vi "Handler - Calib BeginFinish.vi"(8 "error in (no error)":errorcluster, 10 "Finish/Begin (Finish)":bool, 11 "Controller (Host) Data in":T1) -> (0 "error out":errorcluster, 3 "Controller (Host) Data out":T1)   [LabVIEW 2018]
uses:
  cRIO RT Comms/Private Controls/Stream Data.ctl
  cRIO RT Comms/cRIO RT Comms.lvlib
  Top Level/Shared Controls/cRIO State.ctl
  Private Controls/State.ctl
  Controller (Host).lvlib
  Public Controls/APU Select.ctl
  Public Controls/Login Access.ctl
  Private Controls/Controller (Host) Data.ctl
  Top Level/Shared Controls/APU Setup File.ctl
  Public Controls/Test Information.ctl
panel:
  # "Test Information:"
  # "Test Information:"
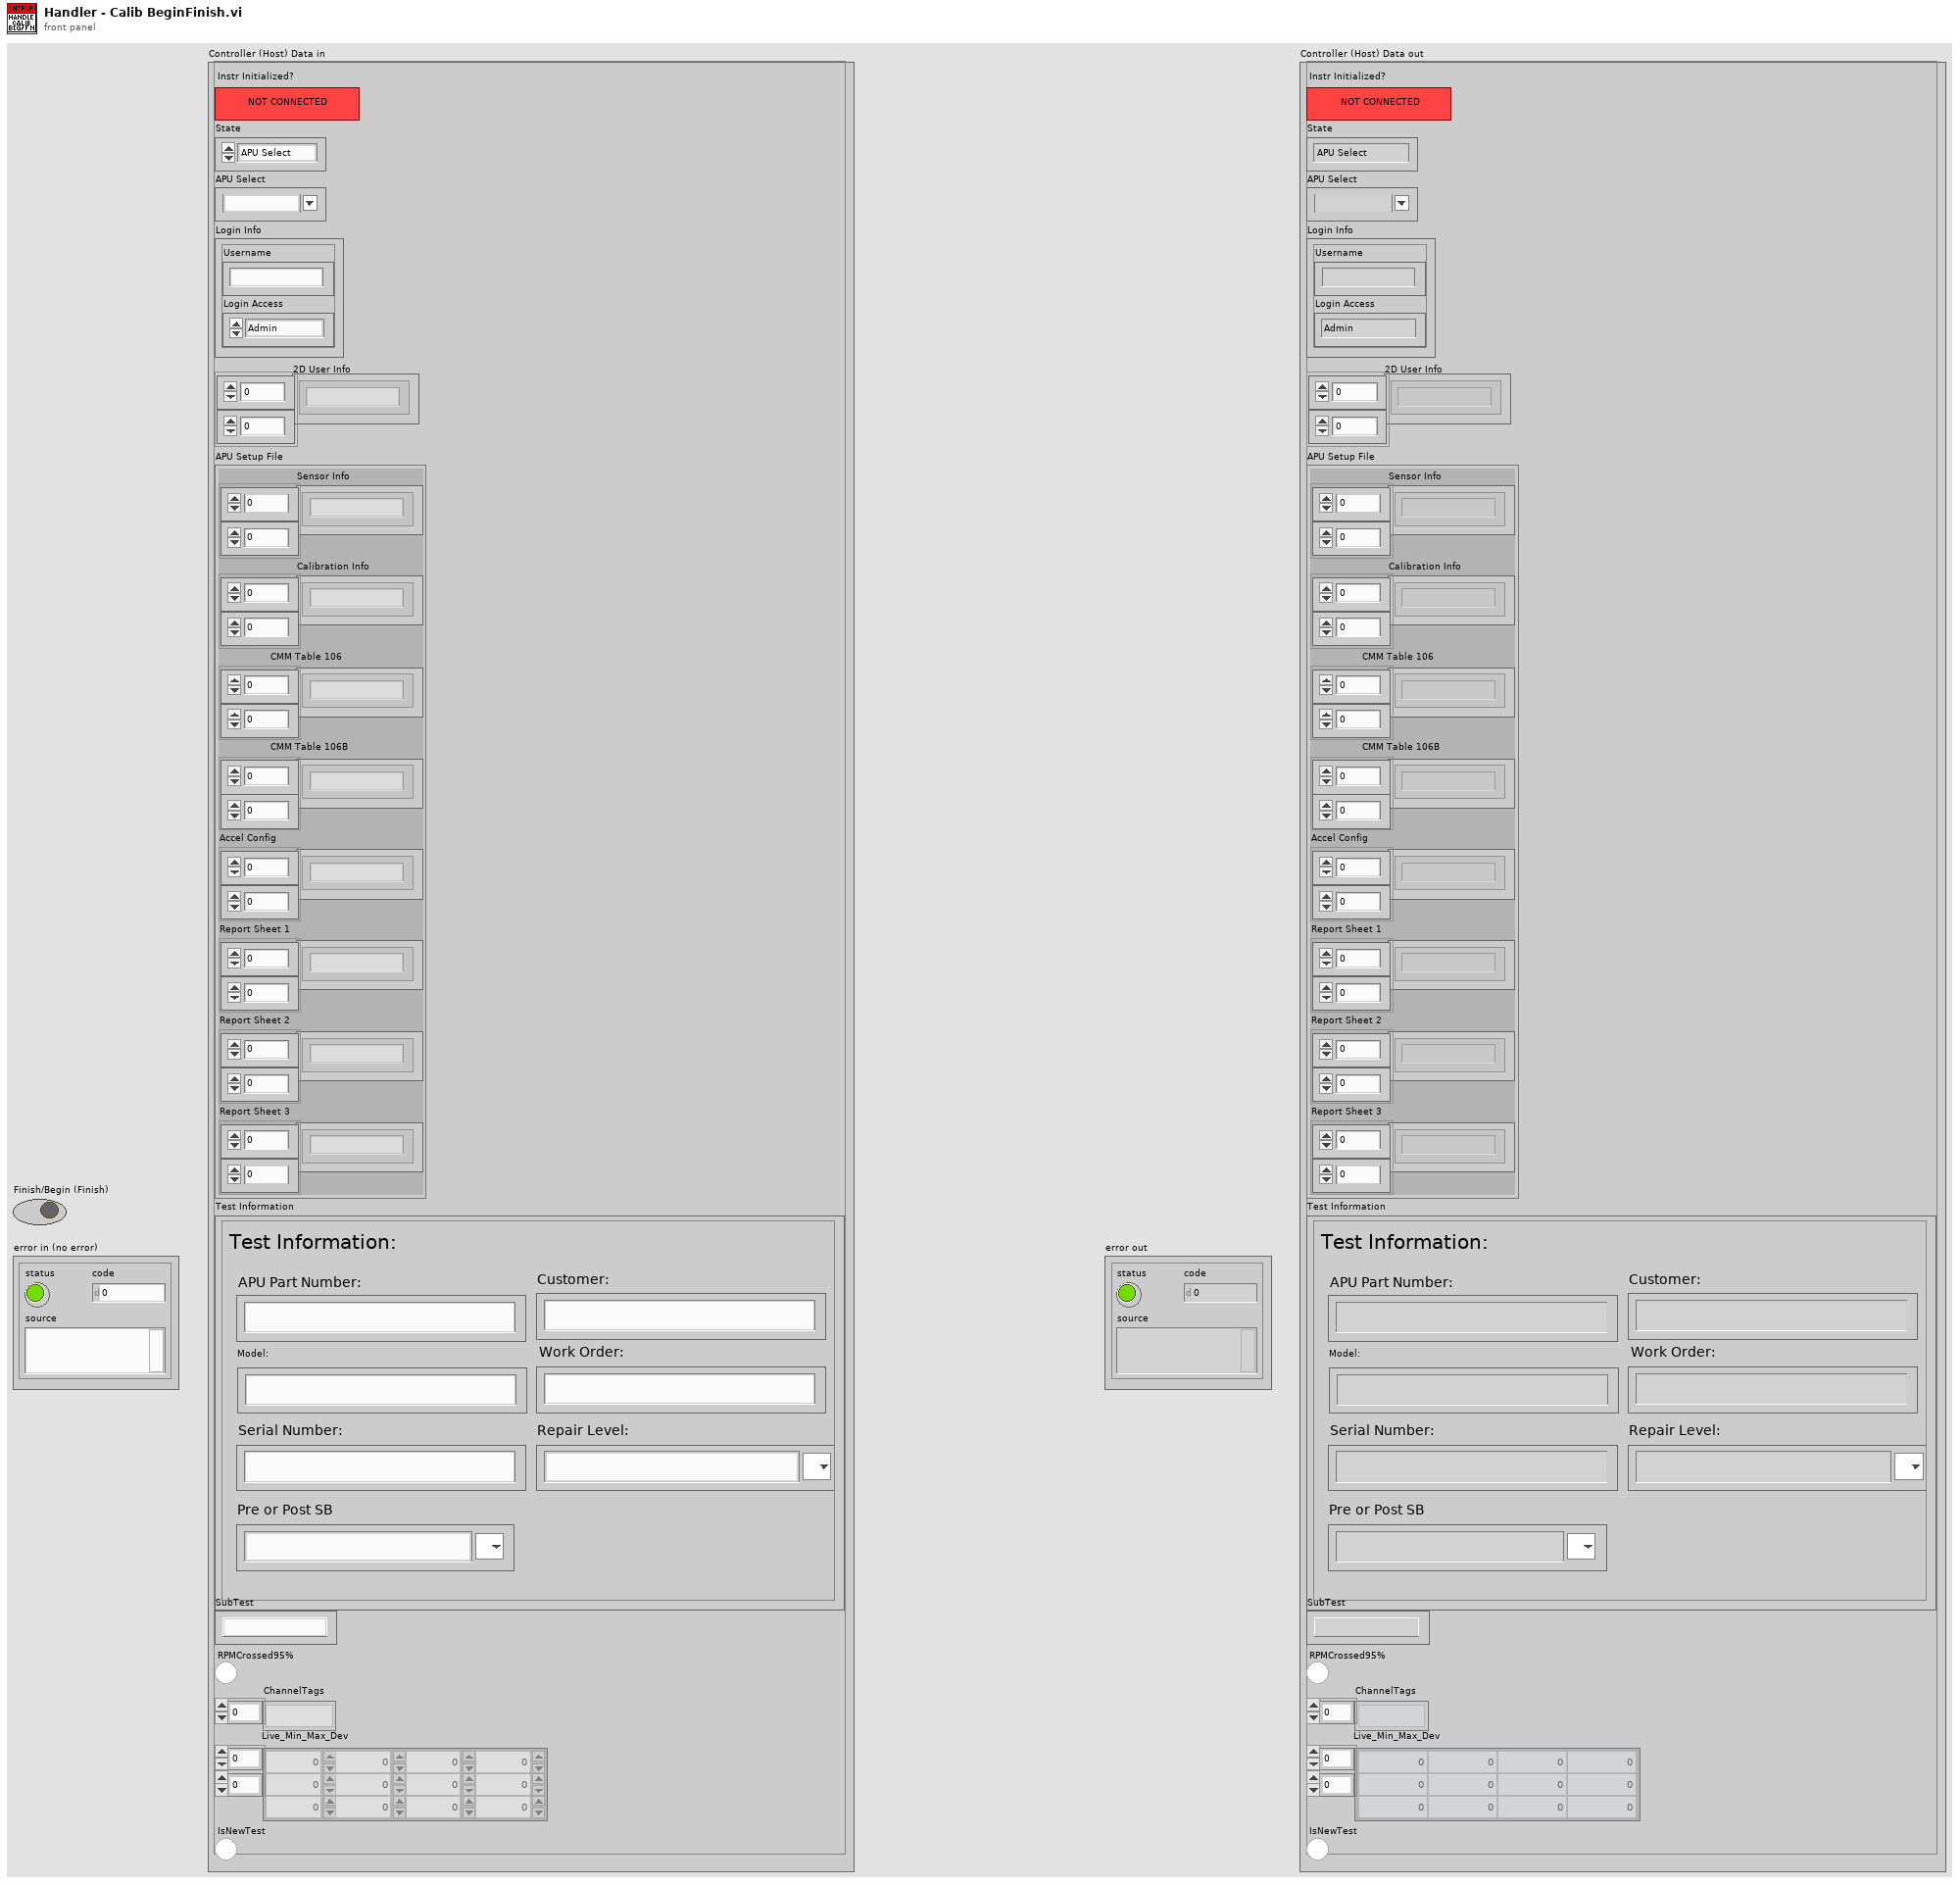
[diagram p1: front panel]
types:
  T1 = typedef "Controller (Host).lvlib/Controller (Host) Data.ctl" = cluster{"Instr Initialized?":bool, "State":T2, "APU Select":T3, "Login Info":cluster{"Username":string, "Login Access":T4}, "2D User Info":string[][], "APU Setup File":T5, "Test Information":T6, "SubTest":string, "RPMCrossed95%":bool, "ChannelTags":string[], "Live_Min_Max_Dev":dbl[][], "IsNewTest":bool}
  T2 = typedef "Controller (Host).lvlib/State.ctl" = enum16{"APU Select", "Operation Select", "SubTests Select", "Calibration", "Testing", "Exit"}
  T3 = typedef "Controller (Host).lvlib/APU Select.ctl" = string
  T4 = typedef "Controller (Host).lvlib/Login Access.ctl" = enum16{"Admin", "Operator", "Guest", ""}
  T5 = typedef "APU Setup File.ctl" = cluster{"Sensor Info":string[][], "Calibration Info":string[][], "CMM Table 106":string[][], "CMM Table 106B ":string[][], "Accel Config":string[][], "Report Sheet 1":string[][], "Report Sheet 2":string[][], "Report Sheet 3":string[][]}
  T6 = typedef "Controller (Host).lvlib/Test Information.ctl" = cluster{"APU Part Number:":string, "Model:":string, "Serial Number:":string, "Customer:":string, "Work Order:":string, "Repair Level:":string, "Pre or Post SB":string}
  T7 = typedef "cRIO RT Comms.lvlib/Stream Data.ctl" = cluster{"Action":string, "Data":variant}
  T8 = typedef "cRIO State.ctl" = enum16{"Waiting for Cal Info", "Idle", "Calibration", "Testing"}
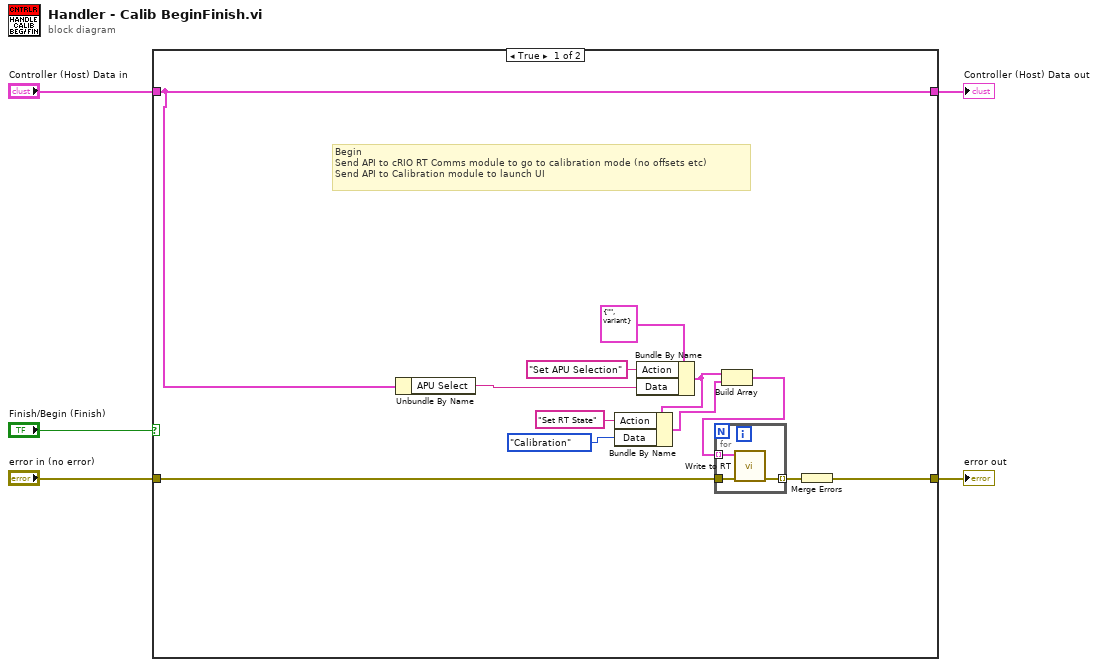
[diagram p0: block diagram]
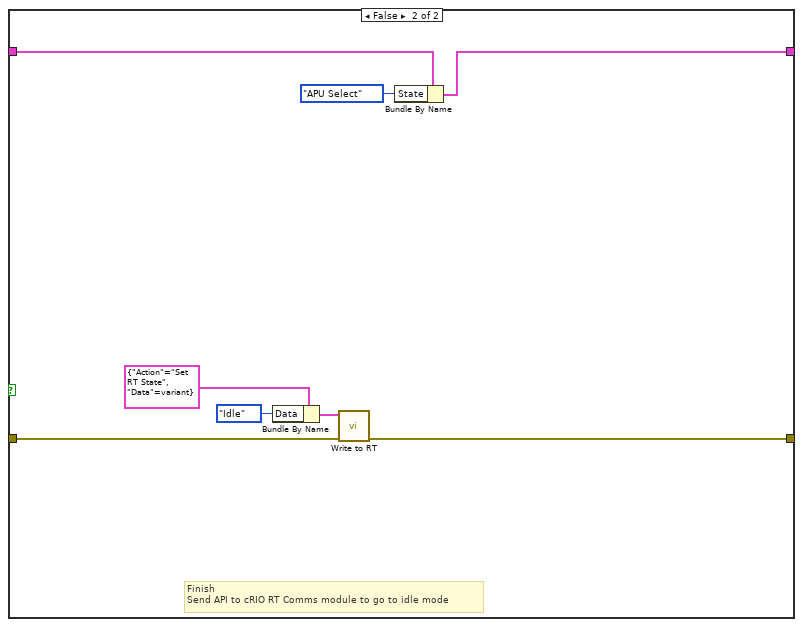
[diagram p2: hidden frame]
diagram:
  n1 = case shown="True" "Finish/Begin (Finish)" {
    tunnel: [w17 w24] -> w2
    tunnel: "error in (no error)" -> [w16 w28]
    tunnel: "Controller (Host) Data in" -> [w15 w23]
    tunnel: [w15 w22] -> w5
    frame True {
      # "Begin\nSend API to cRIO RT Comms module to go to calibration mode (no offsets etc)\nSend API to Calibration module to launch UI"
      n2 = Unbundle By Name(w15) -> ("APU Select"=w8:T3)
      n3 = Bundle By Name(cluster=T7 {"Action"="", "Data"=variant} ("Data to Write"), "Action"="Set APU Selection", "Data"=w8) -> (w7:T7)
      n4 = Bundle By Name(cluster=w7, "Action"="Set RT State", "Data"=cRIO_State."Calibration" ("State")) -> (w9:T7)
      n5 = Build Array(w7, w9) -> (w10:T7[])
      n6 = for {
        tunnel: w10 -> [w20] mode=indexing
        tunnel: w16 -> [w19]
        tunnel: [w18] -> w14 mode=indexing
        n7 = call "Write to RT.vi"("error in (no error)"=w19, "Data to Write"=w20) -> ("error out"=w18:errorcluster)  [unwired: 9 in]
      }
      n8 = Merge Errors(w14) -> (w17:errorcluster)
    }
    frame False {
      # "Finish\nSend API to cRIO RT Comms module to go to idle mode"
      n9 = Bundle By Name(cluster=T7 {"Action"="Set RT State", "Data"=variant} ("Data to Write"), "Data"=cRIO_State."Idle" ("State")) -> (w26:T7)
      n10 = call "Write to RT.vi"("error in (no error)"=w28, "Data to Write"=w26) -> ("error out"=w24:errorcluster)  [unwired: 9 in]
      n11 = Bundle By Name(cluster=w23, "State"=State."APU Select") -> (w22:T1)
    }
  }
  "Controller (Host) Data out" <- w5
  "error out" <- w2
